vi "scale-undef-remover.vi"(10 "Scalenotes Undef":bool[][](array[boolean]), 11 "Scalename undef":string[](array[string])) -> (2 "Scale Notes":bool[][](array[boolean]), 3 "Scale Names":string[](array[string]))   [LabVIEW 2019]
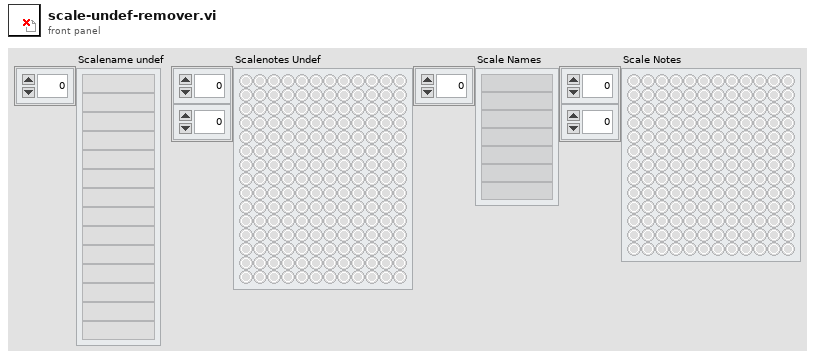
[diagram p1: front panel]
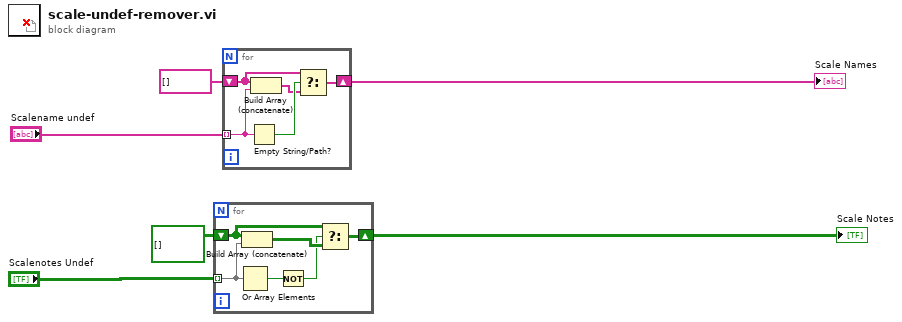
[diagram p0: block diagram]
diagram:
  n1 = for {
    tunnel: "Scalenotes Undef" -> [w9] mode=indexing
    shift-right: [w12] -> w2
    shift-left: bool[][] [] -> [w11]
    n2 = Or Array Elements(Boolean array=w9) -> (logical OR=w8:bool)
    n3 = Build Array (concatenate)(w11, w9) -> (w10:bool[][])
    n4 = Not(x=w8) -> (.not. x?=w7:bool)
    n5 = Select(t=w11, s=w7, f=w10) -> (s? t:f=w12:bool[][])
  }
  "Scale Notes" <- w2
  n6 = for {
    tunnel: "Scalename undef" -> [w14] mode=indexing
    shift-right: [w16] -> w6
    shift-left: string[] [] -> [w15]
    n7 = Empty String/Path?(string/path=w14) -> (empty?=w17:bool)
    n8 = Build Array (concatenate)(w15, w14) -> (w13:string[])
    n9 = Select(t=w15, s=w17, f=w13) -> (s? t:f=w16:string[])
  }
  "Scale Names" <- w6
